vi "Remove Query.vi"(10 "Name":string, 11 "URI in":refnum<class "URI.lvclass">) -> (3 "URI out":refnum<class "URI.lvclass">)   [LabVIEW 2020, in "URI.lvlib" / "URI.lvclass"]
uses:
  URI.lvclass
  URI.lvclass/URI.ctl
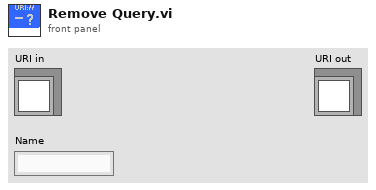
[diagram p1: front panel]
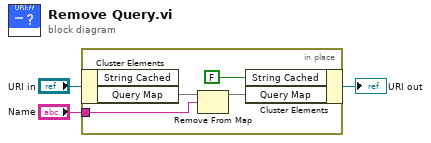
[diagram p0: block diagram]
diagram:
  n1 = in-place {
    in-place-border: "Name" -> [w6]
    n2 = in-place-cluster #1("URI in") -> ("Query Map"=w7:map{string, string})  [unwired: 1 out]
    n3 = Remove From Map(10:w6, 11:w7) -> (3:w5:map{string, string})  [unwired: 2 out]
    n4 = in-place-cluster #1("String Cached"=FALSE, "Query Map"=w5) -> (→"URI out":refnum<class "URI.lvclass">)
  }
